vi "Jason Recursion Binary Tube Search SubVI.vi"(6 "Beginning Tube Number":i32, 7 "End Tube Number":i32, 8 "Clear Pin Task In":refnum<k21>, 9 "Write Pin Task In":refnum<k21>, 10 "Sync Pin Task In":refnum<k21>, 11 "Data Pin Task In":refnum<k21>) -> (0 "Clear Pin Task Out":refnum<k21>, 1 "Write Pin Task Out":refnum<k21>, 2 "Sync Pin Task Out":refnum<k21>, 3 "Data Pin Task Out":refnum<k21>)   [LabVIEW 2020]
uses:
  <vilib>/numeric/Random Number (Range) DBL.vi
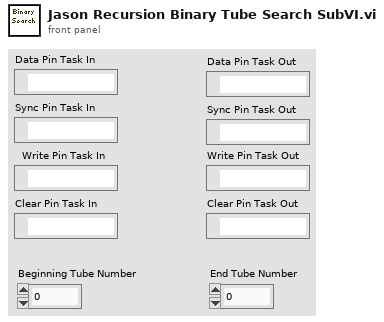
[diagram p1: front panel]
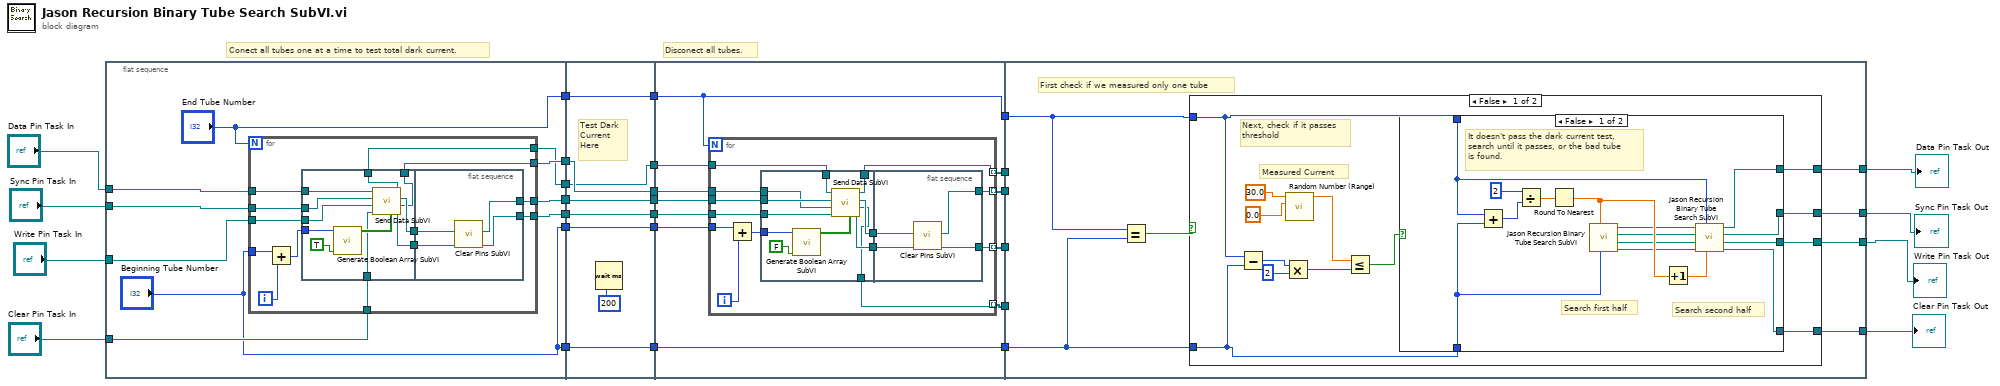
[diagram p0: block diagram]
diagram:
  # "Disconect all tubes."
  # "Conect all tubes one at a time to test total dark current."
  n1 = flat-sequence {
    tunnel: "Data Pin Task In" -> [w38]
    tunnel: "Sync Pin Task In" -> [w37]
    tunnel: "Write Pin Task In" -> [w36]
    tunnel: "Clear Pin Task In" -> [w35]
    tunnel: ["End Tube Number"] -> w23
    tunnel: [w33] -> w21
    tunnel: [w32] -> w19
    tunnel: [w31] -> w17
    tunnel: [w30] -> w15
    tunnel: ["Beginning Tube Number"] -> w12
    tunnel: ["Beginning Tube Number"] -> w9
    tunnel: [w73] -> w24
    tunnel: w23 -> [w73]
    tunnel: [w72] -> w22
    tunnel: w21 -> [w72]
    tunnel: [w71] -> w20
    tunnel: w19 -> [w71]
    tunnel: [w70] -> w18
    tunnel: w17 -> [w70]
    tunnel: [w69] -> w16
    tunnel: w15 -> [w69]
    tunnel: [w68] -> w13
    tunnel: w12 -> [w68]
    tunnel: [w67] -> w10
    tunnel: w9 -> [w67]
    tunnel: w24 -> [w81]
    tunnel: w22 -> [w85]
    tunnel: w20 -> [w84]
    tunnel: w18 -> [w83]
    tunnel: w16 -> [w82]
    tunnel: [w81] -> w14
    tunnel: w13 -> [w80]
    tunnel: [w79] -> w11
    tunnel: w10 -> [w79]
    tunnel: [w78] -> w8
    tunnel: [w77] -> w7
    tunnel: [w76] -> w6
    tunnel: [w75] -> w5
    tunnel: w14 -> [w119]
    tunnel: w11 -> [w118]
    tunnel: w8 -> [_]
    tunnel: w7 -> [_]
    tunnel: w6 -> [_]
    tunnel: w5 -> [_]
    tunnel: [w117] -> w4
    tunnel: [w116] -> w3
    tunnel: [w115] -> w2
    tunnel: [w114] -> w1
    frame #0 {
      n2 = for {
        N: "End Tube Number" -> [_]
        tunnel: w38 -> [w51]
        tunnel: w37 -> [w50]
        tunnel: w36 -> [w49]
        tunnel: w35 -> [w48]
        tunnel: [w45] -> w33
        tunnel: [w44] -> w32
        tunnel: [w43] -> w31
        tunnel: [w42] -> w30
        tunnel: "Beginning Tube Number" -> [w39]
        i -> [w40]
        n3 = Add(x=w39, y=w40) -> (x+y=w41:i32)
        n4 = flat-sequence {
          tunnel: w41 -> [w60]
          tunnel: w51 -> [w59]
          tunnel: w50 -> [w58]
          tunnel: w49 -> [w57]
          tunnel: w48 -> [w56]
          tunnel: [w55] -> w47
          tunnel: [w54] -> w46
          tunnel: [w53] -> w43
          tunnel: [w52] -> w42
          tunnel: w47 -> [w66]
          tunnel: w46 -> [w65]
          tunnel: [w64] -> w45
          tunnel: [w63] -> w44
          frame #0 {
            n5 = call "Generate Boolean Array SubVI.vi"("Activate: 1\nDeactivate: 0"=TRUE, "Tube"=w60) -> ("Boolean array"=w61:bool[])  [unwired: 9 in]
            n6 = call "Send Data SubVI.vi"("Data Pin Task In"=w59, "Sync Pin Task In"=w58, "Write Pin Task In"=w57, "Clear Pin Task In"=w56, "Data"=w61) -> ("Data Pin Task Out"=w52:refnum<k21>, "Sync Pin Task Out"=w55:refnum<k21>, "Write Pin Task Out"=w53:refnum<k21>, "Clear Pin Task Out"=w54:refnum<k21>)  [unwired: 1 in]
          }
          frame #1 {
            n7 = call "Clear Pins SubVI.vi"("Clear Pin Task In"=w65, "Sync Pin Task In"=w66) -> ("Clear Pin Task Out"=w63:refnum<k21>, "Sync Pin Task Out"=w64:refnum<k21>)  [unwired: 8 in]
          }
        }
      }
    }
    frame #1 {
      # "Test Dark \nCurrent \nHere"
      n8 = Wait (ms)(milliseconds to wait=u32 200) -> ()  [unwired: 1 out]
    }
    frame #2 {
      n9 = for {
        N: w81 -> [_]
        tunnel: w85 -> [w96]
        tunnel: w84 -> [w95]
        tunnel: w83 -> [w94]
        tunnel: w82 -> [w93]
        tunnel: w80 -> [w90]
        tunnel: [w89] -> w78 mode=indexing
        tunnel: [w88] -> w77 mode=indexing
        tunnel: [w87] -> w76 mode=indexing
        tunnel: [w86] -> w75 mode=indexing
        i -> [w91]
        n10 = Add(x=w90, y=w91) -> (x+y=w92:i32)
        n11 = flat-sequence {
          tunnel: w92 -> [w107]
          tunnel: [w106] -> w98
          tunnel: [w105] -> w97
          tunnel: w96 -> [w104]
          tunnel: w95 -> [w103]
          tunnel: w94 -> [w102]
          tunnel: w93 -> [w101]
          tunnel: [w100] -> w89
          tunnel: [w99] -> w87
          tunnel: w98 -> [w113]
          tunnel: w97 -> [w112]
          tunnel: [w111] -> w88
          tunnel: [w110] -> w86
          frame #0 {
            n12 = call "Generate Boolean Array SubVI.vi"("Activate: 1\nDeactivate: 0"=FALSE, "Tube"=w107) -> ("Boolean array"=w108:bool[])  [unwired: 9 in]
            n13 = call "Send Data SubVI.vi"("Data Pin Task In"=w101, "Sync Pin Task In"=w104, "Write Pin Task In"=w102, "Clear Pin Task In"=w103, "Data"=w108) -> ("Data Pin Task Out"=w100:refnum<k21>, "Sync Pin Task Out"=w106:refnum<k21>, "Write Pin Task Out"=w99:refnum<k21>, "Clear Pin Task Out"=w105:refnum<k21>)  [unwired: 1 in]
          }
          frame #1 {
            n14 = call "Clear Pins SubVI.vi"("Clear Pin Task In"=w112, "Sync Pin Task In"=w113) -> ("Clear Pin Task Out"=w110:refnum<k21>, "Sync Pin Task Out"=w111:refnum<k21>)  [unwired: 8 in]
          }
        }
      }
    }
    frame #3 {
      # "First check if we measured only one tube"
      n15 = Equal?(x=w119, y=w118) -> (x = y?=w120:bool)
      n16 = case shown="False" w120 {
        tunnel: w119 -> [w126 _]
        tunnel: w118 -> [w125 _]
        tunnel: [w124 _] -> w117
        tunnel: [w123 _] -> w116
        tunnel: [w122 _] -> w115
        tunnel: [w121 _] -> w114
        frame False {
          # "Next, check if it passes\nthreshold"
          # "Measured Current"
          n17 = Subtract(x=w126, y=w125) -> (x-y=w128:i32)
          n18 = Multiply(x=w128, y=2) -> (x*y=w133:i32)
          n19 = call-poly <vilib>:"Random Number (Range).vi"("lower bound (0)"=0.0, "upper bound (100)"=30.0) -> ("number"=w132:dbl)  [unwired: 9 in]
          n20 = Less Or Equal?(x=w132, y=w133) -> (x <= y?=w127:bool)
          n21 = case shown="False" w127 {
            tunnel: w126 -> [w144 _]
            tunnel: w125 -> [w146 _]
            tunnel: [w137 _] -> w124
            tunnel: [w136 _] -> w123
            tunnel: [w135 _] -> w122
            tunnel: [w134 _] -> w121
            frame False {
              # "Search second half"
              # "Search first half"
              # "It doesn't pass the dark current test,\nsearch until it passes, or the bad tube\nis found."
              n22 = Add(x=w144, y=w146) -> (x+y=w147:i32)
              n23 = Divide(x=2, y=w147) -> (x/y=w148:dbl)
              n24 = Round To Nearest(number=w148) -> (nearest integer value=w142:dbl)
              n25 = call "Jason Recursion Binary Tube Search SubVI.vi"("Beginning Tube Number"=w146, "End Tube Number"=w142) -> ("Clear Pin Task Out"=w138:refnum<k21>, "Write Pin Task Out"=w139:refnum<k21>, "Sync Pin Task Out"=w140:refnum<k21>, "Data Pin Task Out"=w141:refnum<k21>)  [unwired: 6 in]
              n26 = Increment(x=w142) -> (x+1=w143:dbl)
              n27 = call "Jason Recursion Binary Tube Search SubVI.vi"("Beginning Tube Number"=w143, "End Tube Number"=w144, "Clear Pin Task In"=w138, "Write Pin Task In"=w139, "Sync Pin Task In"=w140, "Data Pin Task In"=w141) -> ("Clear Pin Task Out"=w134:refnum<k21>, "Write Pin Task Out"=w135:refnum<k21>, "Sync Pin Task Out"=w136:refnum<k21>, "Data Pin Task Out"=w137:refnum<k21>)  [unwired: 2 in]
            }
            frame True {
              # "It passes the dark current test, write the values to the database"
            }
          }
        }
        frame True {
          # "Yes, we previously only tested one 1ube, write this value to the database"
        }
      }
    }
  }
  "Clear Pin Task Out" <- w1
  "Data Pin Task Out" <- w4
  "Write Pin Task Out" <- w2
  "Sync Pin Task Out" <- w3
